vi "Intersection and Difference.vi"(8 "error in (no error)":errorcluster, 10 "Cube A":refnum<class "Cube.lvclass">, 11 "Cube B in":refnum<class "Cube.lvclass">) -> (0 "error out":errorcluster, 1 "Intersection":refnum<class "Cube.lvclass">, 2 "Difference":refnum<class "Cube.lvclass">[](array[class]), 3 "Cube B out":refnum<class "Cube.lvclass">, 4 "Intersection Found?":bool)   [LabVIEW 2019, in "22.lvlib" / "Cube.lvclass"]
uses:
  Cube.lvclass
  Cube.lvclass/Cube.ctl
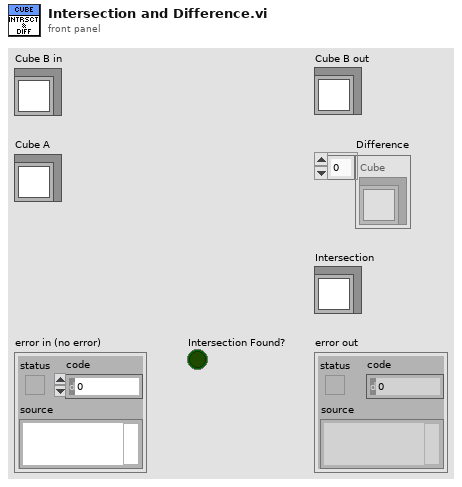
[diagram p1: front panel]
types:
  T1 = cluster{"xmin":i64, "xmax":i64, "ymin":i64, "ymax":i64, "zmin":i64, "zmax":i64}
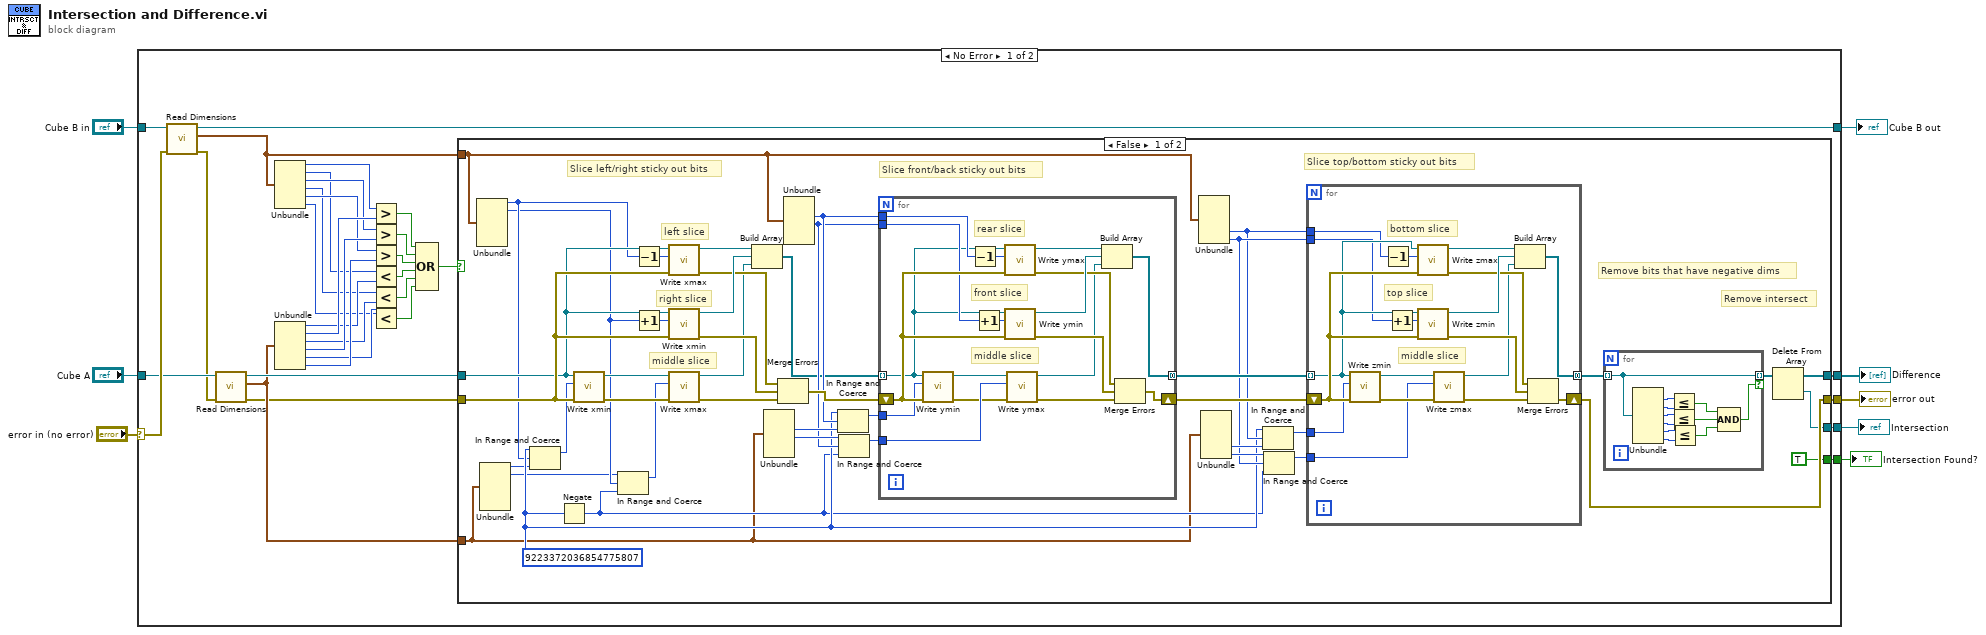
[diagram p0: block diagram]
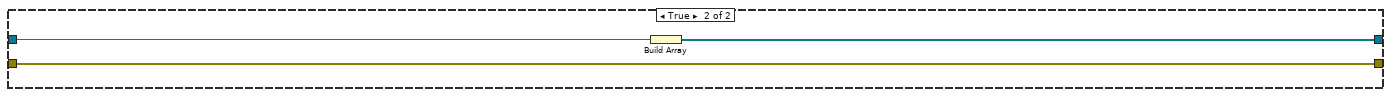
[diagram p2: hidden frame]
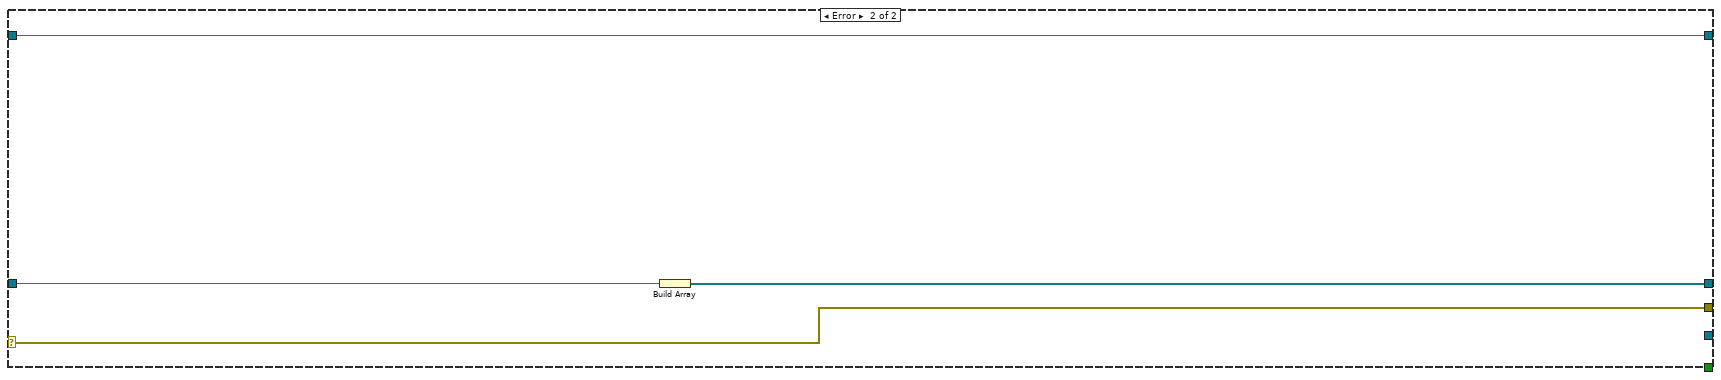
[diagram p3: hidden frame]
diagram:
  n1 = case shown="No Error" "error in (no error)" {
    selector: "error in (no error)" -> [w39 w138]
    tunnel: [w38 w138] -> w7
    tunnel: "Cube B in" -> [w40 w137]
    tunnel: "Cube A" -> [w36 w136]
    tunnel: [w34 w135] -> w4
    tunnel: [w35 w137] -> w3
    tunnel: [w10 _] -> w2
    tunnel: [w9 _] -> w1
    frame No Error {
      n2 = call-dynamic "Read Dimensions.vi"("error in (no error)"=w39, "Cube in"=w40) -> ("error out"=w19:errorcluster, "Dimensions"=w33:T1, "Cube out"=w35:refnum<class "Cube.lvclass">)  [unwired: 7 in]
      n3 = call-dynamic "Read Dimensions.vi"("error in (no error)"=w19, "Cube in"=w36) -> ("error out"=w18:errorcluster, "Dimensions"=w32:T1, "Cube out"=w37:refnum<class "Cube.lvclass">)  [unwired: 7 in]
      n4 = Unbundle(w33) -> ("xmin"=w31:i64, "xmax"=w25:i64, "ymin"=w29:i64, "ymax"=w23:i64, "zmin"=w27:i64, "zmax"=w20:i64)
      n5 = Unbundle(w32) -> ("xmin"=w24:i64, "xmax"=w30:i64, "ymin"=w22:i64, "ymax"=w28:i64, "zmin"=w21:i64, "zmax"=w26:i64)
      n6 = Greater?(x=w31, y=w30) -> (0:w17:bool)
      n7 = Greater?(x=w29, y=w28) -> (0:w16:bool)
      n8 = Greater?(x=w27, y=w26) -> (0:w14:bool)
      n9 = Less?(x=w25, y=w24) -> (x < y?=w13:bool)
      n10 = Less?(x=w23, y=w22) -> (x < y?=w12:bool)
      n11 = Less?(x=w20, y=w21) -> (x < y?=w11:bool)
      n12 = Compound Arithmetic op=OR(w17, w16, w14, w13, w12, w11) -> (w15:bool)
      n13 = case shown="False" w15 {
        tunnel: w18 -> [w84 w132]
        tunnel: w33 -> [w51 _]
        tunnel: [w73 w132] -> w38
        tunnel: w37 -> [w72 w134]
        tunnel: w32 -> [w48 _]
        tunnel: [w44 w133] -> w34
        tunnel: [w42 _] -> w10
        tunnel: [TRUE _] -> w9
        frame False {
          w55 = i64 9223372036854775807 ("upper limit")
          # "Remove bits that have negative dims"
          # "Slice top/bottom sticky out bits"
          # "Slice front/back sticky out bits"
          # "Slice left/right sticky out bits"
          # "Remove intersect"
          # "middle slice"
          # "right slice"
          # "left slice"
          n14 = Unbundle(w51) -> ("xmin"=w50:i64, "xmax"=w49:i64)  [unwired: 4 out]
          n15 = Unbundle(w48) -> ("xmin"=w47:i64, "xmax"=w46:i64)  [unwired: 4 out]
          n16 = In Range and Coerce(upper limit=w55, x=w50, lower limit=w47) -> (coerced(x)=w71:i64)  [unwired: 1 out]
          n17 = Negate(x=w55) -> (-x=w54:i64)
          n18 = call-dynamic "Write xmin.vi"("error in (no error)"=w84, "xmin"=w71, "Cube in"=w72) -> ("error out"=w81:errorcluster, "Cube out"=w80:refnum<class "Cube.lvclass">)  [unwired: 7 in]
          n19 = In Range and Coerce(upper limit=w46, x=w49, lower limit=w54) -> (coerced(x)=w70:i64)  [unwired: 1 out]
          n20 = Decrement(x=w50) -> (x-1=w83:i64)
          n21 = Increment(x=w49) -> (x+1=w82:i64)
          n22 = call-dynamic "Write xmax.vi"("error in (no error)"=w84, "xmax"=w83, "Cube in"=w72) -> ("error out"=w77:errorcluster, "Cube out"=w79:refnum<class "Cube.lvclass">)  [unwired: 7 in]
          n23 = call-dynamic "Write xmin.vi"("error in (no error)"=w84, "xmin"=w82, "Cube in"=w72) -> ("error out"=w76:errorcluster, "Cube out"=w78:refnum<class "Cube.lvclass">)  [unwired: 7 in]
          n24 = call-dynamic "Write xmax.vi"("error in (no error)"=w81, "xmax"=w70, "Cube in"=w80) -> ("error out"=w75:errorcluster, "Cube out"=w63:refnum<class "Cube.lvclass">)  [unwired: 7 in]
          n25 = Build Array(w79, w78, w63) -> (w62:refnum<class "Cube.lvclass">[])
          n26 = Unbundle(w48) -> ("ymin"=w68:i64, "ymax"=w66:i64)  [unwired: 4 out]
          n27 = Merge Errors(w77, w76, w75) -> (w74:errorcluster)
          n28 = Unbundle(w51) -> ("ymin"=w69:i64, "ymax"=w65:i64)  [unwired: 4 out]
          n29 = In Range and Coerce(upper limit=w55, x=w69, lower limit=w68) -> (coerced(x)=w67:i64)  [unwired: 1 out]
          n30 = In Range and Coerce(upper limit=w66, x=w65, lower limit=w54) -> (coerced(x)=w64:i64)  [unwired: 1 out]
          n31 = for {
            tunnel: w69 -> [w119]
            tunnel: w67 -> [w118]
            tunnel: w65 -> [w117]
            tunnel: w64 -> [w116]
            tunnel: w62 -> [w115] mode=indexing
            tunnel: [w103] -> w60 mode=concatenating
            shift-right: [w104] -> w61
            shift-left: w74 -> [w120]
            # "middle slice"
            # "front slice"
            # "rear slice"
            n32 = call-dynamic "Write ymin.vi"("error in (no error)"=w120, "ymin"=w118, "Cube in"=w115) -> ("error out"=w111:errorcluster, "Cube out"=w112:refnum<class "Cube.lvclass">)  [unwired: 7 in]
            n33 = Decrement(x=w119) -> (x-1=w114:i64)
            n34 = Increment(x=w117) -> (x+1=w113:i64)
            n35 = call-dynamic "Write ymax.vi"("error in (no error)"=w120, "ymax"=w114, "Cube in"=w115) -> ("error out"=w106:errorcluster, "Cube out"=w110:refnum<class "Cube.lvclass">)  [unwired: 7 in]
            n36 = call-dynamic "Write ymin.vi"("error in (no error)"=w120, "ymin"=w113, "Cube in"=w115) -> ("error out"=w107:errorcluster, "Cube out"=w109:refnum<class "Cube.lvclass">)  [unwired: 7 in]
            n37 = call-dynamic "Write ymax.vi"("error in (no error)"=w111, "ymax"=w116, "Cube in"=w112) -> ("error out"=w108:errorcluster, "Cube out"=w105:refnum<class "Cube.lvclass">)  [unwired: 7 in]
            n38 = Build Array(w110, w109, w105) -> (w103:refnum<class "Cube.lvclass">[])
            n39 = Merge Errors(w106, w107, w108) -> (w104:errorcluster)
          }
          n40 = Unbundle(w51) -> ("zmin"=w56:i64, "zmax"=w57:i64)  [unwired: 4 out]
          n41 = Unbundle(w48) -> ("zmin"=w59:i64, "zmax"=w58:i64)  [unwired: 4 out]
          n42 = In Range and Coerce(upper limit=w55, x=w56, lower limit=w59) -> (coerced(x)=w53:i64)  [unwired: 1 out]
          n43 = In Range and Coerce(upper limit=w58, x=w57, lower limit=w54) -> (coerced(x)=w52:i64)  [unwired: 1 out]
          n44 = for {
            tunnel: [w101] -> w45 mode=concatenating
            tunnel: w60 -> [w90] mode=indexing
            tunnel: w57 -> [w89]
            tunnel: w56 -> [w88]
            shift-right: [w102] -> w73
            shift-left: w61 -> [w92]
            tunnel: w53 -> [w87]
            tunnel: w52 -> [w86]
            # "middle slice"
            # "top slice"
            # "bottom slice"
            n45 = call-dynamic "Write zmin.vi"("error in (no error)"=w92, "zmin"=w87, "Cube in"=w90) -> ("error out"=w93:errorcluster, "Cube out"=w94:refnum<class "Cube.lvclass">)  [unwired: 7 in]
            n46 = Decrement(x=w88) -> (x-1=w100:i64)
            n47 = Increment(x=w89) -> (x+1=w99:i64)
            n48 = call-dynamic "Write zmax.vi"("error in (no error)"=w92, "zmax"=w100, "Cube in"=w90) -> ("error out"=w95:errorcluster, "Cube out"=w98:refnum<class "Cube.lvclass">)  [unwired: 7 in]
            n49 = call-dynamic "Write zmin.vi"("error in (no error)"=w92, "zmin"=w99, "Cube in"=w90) -> ("error out"=w96:errorcluster, "Cube out"=w97:refnum<class "Cube.lvclass">)  [unwired: 7 in]
            n50 = call-dynamic "Write zmax.vi"("error in (no error)"=w93, "zmax"=w86, "Cube in"=w94) -> ("error out"=w91:errorcluster, "Cube out"=w85:refnum<class "Cube.lvclass">)  [unwired: 7 in]
            n51 = Build Array(w98, w97, w85) -> (w101:refnum<class "Cube.lvclass">[])
            n52 = Merge Errors(w95, w96, w91) -> (w102:errorcluster)
          }
          n53 = for {
            tunnel: w45 -> [w128] mode=indexing
            tunnel: [w128] -> w43 mode=indexing if=w123
            n54 = Unbundle(w128) -> (w125:i64, w124:i64, w127:i64, w126:i64, w130:i64, w129:i64)  [unwired: 1 out]
            n55 = Less Or Equal?(x=w125, y=w124) -> (x <= y?=w121:bool)
            n56 = Less Or Equal?(x=w127, y=w126) -> (x <= y?=w122:bool)
            n57 = Less Or Equal?(x=w130, y=w129) -> (x <= y?=w131:bool)
            n58 = Compound Arithmetic op=AND(w121, w122, w131) -> (w123:bool)
          }
          n59 = Delete From Array(array=w43) -> (deleted portion=w42:refnum<class "Cube.lvclass">, array with subset deleted=w44:refnum<class "Cube.lvclass">[])  [unwired: 2 in]
        }
        frame True {
          n60 = Build Array(w134) -> (w133:refnum<class "Cube.lvclass">[])
        }
      }
    }
    frame Error {
      n61 = Build Array(w136) -> (w135:refnum<class "Cube.lvclass">[])
    }
  }
  "error out" <- w7
  "Difference" <- w4
  "Cube B out" <- w3
  "Intersection" <- w2
  "Intersection Found?" <- w1
